vi "Get Connection Properties.vi"(8 "error in (no error)":errorcluster, 11 "Device Item Ref in":T1 format="%.0x") -> (0 "error out":errorcluster, 2 "AutoSelect":T2, 3 "Item Ref out":T1 format="%.0x")   [LabVIEW 2015, in "Chassis TimeSync System Explorer.lvlib"]
uses:
  Chassis TimeSync System Explorer.lvlib
  Shared/Connection Settings.ctl
  Shared/Mode.ctl
  Shared/External Pin.ctl
  Shared/Routes.ctl
  Shared/Route.ctl
  <vilib>/NI Veristand/Custom Device API/Custom Device Item Ref.ctl
  Shared/Constants.vi
  <vilib>/NI Veristand/Custom Device API/Get Item Property (U16).vi
  <vilib>/NI Veristand/Custom Device API/Get Item Property (Boolean).vi
  Shared/Chassis TimeSync Shared.lvlib
  <vilib>/NI Veristand/Custom Device API/Custom Device API.lvlib
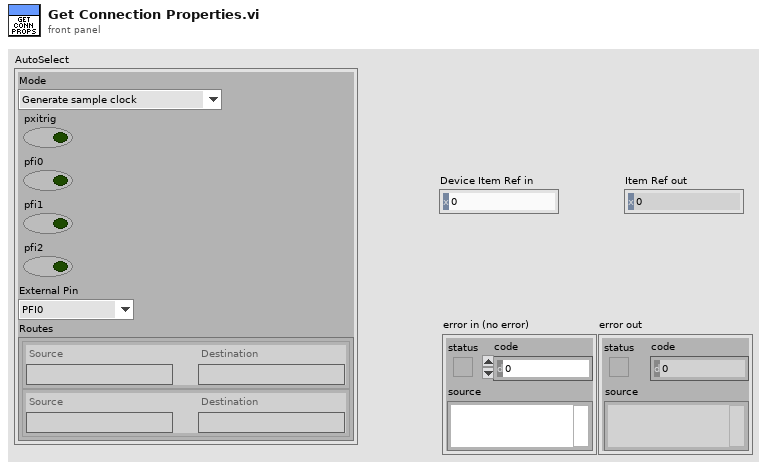
[diagram p1: front panel]
types:
  T1 = typedef "Custom Device API.lvlib/Custom Device Item Ref.ctl" = u64
  T2 = typedef "Chassis TimeSync Shared.lvlib/Connection Settings.ctl" = cluster{"Mode":T3, "pxitrig":bool, "pfi0":bool, "pfi1":bool, "pfi2":bool, "External Pin":T4, "Routes":T5}
  T3 = typedef "Chassis TimeSync Shared.lvlib/Mode.ctl" = enum16{"Generate sample clock", "Route sample clock out of chassis", "Route sample clock into chassis", "Custom routes"}
  T4 = typedef "Chassis TimeSync Shared.lvlib/External Pin.ctl" = enum16{"PFI0", "PFI1", "PFI2"}
  T5 = typedef "Chassis TimeSync Shared.lvlib/Routes.ctl" = T6[]
  T6 = typedef "Chassis TimeSync Shared.lvlib/Route.ctl" = cluster{"Source":string, "Destination":string}
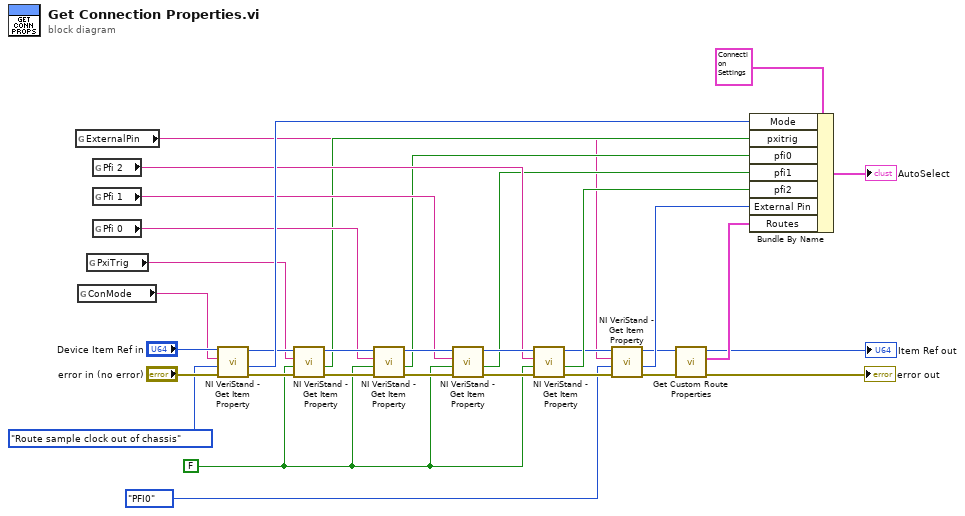
[diagram p0: block diagram]
diagram:
  w15 = FALSE ("pxitrig")
  n1 = global read "Constants.vi" "ExternalPin"() -> (w8:string)
  n2 = global read "Constants.vi" "ConMode"() -> (w30:string)
  n3 = global read "Constants.vi" "PxiTrig"() -> (w25:string)
  n4 = global read "Constants.vi" "Pfi 2"() -> (w16:string)
  n5 = global read "Constants.vi" "Pfi 1"() -> (w19:string)
  n6 = global read "Constants.vi" "Pfi 0"() -> (w22:string)
  n7 = call-poly <vilib>:"NI VeriStand - Get Item Property.vi"("error in (no error)"="error in (no error)", "Default Value"=Mode."Route sample clock out of chassis" ("Mode"), "Property Name"=w30, "Item Ref in"="Device Item Ref in") -> ("error out"=w26:errorcluster, "Value"=w28:u16, "Item Ref out"=w27:T1)  [unwired: 4 in, 1 out]
  n8 = call-poly <vilib>:"NI VeriStand - Get Item Property.vi"("error in (no error)"=w26, "Default Value"=w15, "Property Name"=w25, "Item Ref in"=w27) -> ("error out"=w23:errorcluster, "Value"=w14:bool, "Item Ref out"=w24:T1)  [unwired: 4 in, 1 out]
  n9 = call-poly <vilib>:"NI VeriStand - Get Item Property.vi"("error in (no error)"=w23, "Default Value"=w15, "Property Name"=w22, "Item Ref in"=w24) -> ("error out"=w20:errorcluster, "Value"=w13:bool, "Item Ref out"=w21:T1)  [unwired: 4 in, 1 out]
  n10 = call-poly <vilib>:"NI VeriStand - Get Item Property.vi"("error in (no error)"=w20, "Default Value"=w15, "Property Name"=w19, "Item Ref in"=w21) -> ("error out"=w17:errorcluster, "Value"=w12:bool, "Item Ref out"=w18:T1)  [unwired: 4 in, 1 out]
  n11 = call-poly <vilib>:"NI VeriStand - Get Item Property.vi"("error in (no error)"=w17, "Default Value"=w15, "Property Name"=w16, "Item Ref in"=w18) -> ("error out"=w10:errorcluster, "Value"=w11:bool, "Item Ref out"=w9:T1)  [unwired: 4 in, 1 out]
  n12 = call-poly <vilib>:"NI VeriStand - Get Item Property.vi"("error in (no error)"=w10, "Default Value"=External_Pin."PFI0" ("External Pin"), "Property Name"=w8, "Item Ref in"=w9) -> ("error out"=w5:errorcluster, "Value"=w6:u16, "Item Ref out"=w4:T1)  [unwired: 4 in, 1 out]
  n13 = call "Get Custom Route Properties.vi"("error in (no error)"=w5, "Item Ref in"=w4) -> ("error out"=→"error out":errorcluster, "Routes"=w3:T5, "Item Ref out"=→"Item Ref out":T1)  [unwired: 7 in]
  n14 = Bundle By Name(cluster=T2 {"Mode"=enum."Generate sample clock", "pxitrig"=FALSE, "pfi0"=TRUE, "pfi1"=TRUE, "pfi2"=TRUE, "External Pin"=enum."PFI0", "Routes"=[]}, "Mode"=w28, "pxitrig"=w14, "pfi0"=w13, "pfi1"=w12, "pfi2"=w11, "External Pin"=w6, "Routes"=w3) -> (→"AutoSelect":T2)
